vi "_s_Bronkhorst Serial Read Flows.vi"(6 "Delay Time (s)":dbl=0.1, 7 "Comunicaciones":T2={"Flujo_1"="COM1", "Brk1"=FALSE, "Flujo_2"="COM2", "Brk2"=FALSE, "Flujo_3"="COM3", "Brk3"=FALSE, "Flujo_4"="COM4", "Brk4"=FALSE, "Eurothe"="COM5", "Eurot"=FALSE, "Balanza"="ASRL6::INSTR", "Bal"=FALSE, "eValPos"="ASRL6::INSTR", "eVal"=FALSE, "flowbus"="ASRL6::INSTR", "fb"=FALSE}, 8 "error in (no error)":errorcluster) -> (0 "error out":errorcluster, 2 "Dispositivos":T1=[["3", "NO", "M0000013", "Air", "1", "ln/mn", "0", "0"], ["4", "NO", "M0000014", "Air", "1", "ln/mn", "0", "0"], ["5", "NO", "M0000015", "Air", "1", "ln/mn", "0", "0"], ["6", "NO", "M0000016", "Air", "1", "ln/mn", "0", "0"], ["7", "NO", "M0000017", "Air", "1", "ln/mn", "0", "0"], ["8", "NO", "M0000018", "Air", "1", "ln/mn", "0", "0"], ["9", "NO", "M0000019", "Air", "1", "ln/mn", "0", "0"], ["10", "NO", "M0000020", "Air", "1", "ln/mn", "0", "0"], ["11", "NO", "M0000021", "Air", "1", "ln/mn", "0", "0"]] caption="MassFlowControllers")   [LabVIEW 2013]
uses:
  Controles/P2018 Com Control.ctl
  _s_TablaBronkhorst.ctl
  _s_Bronkhorst Control.ctl
  P2022 TB INCAR GLOBALES.vi
panel:
  out "Num. of nodes":u32=6
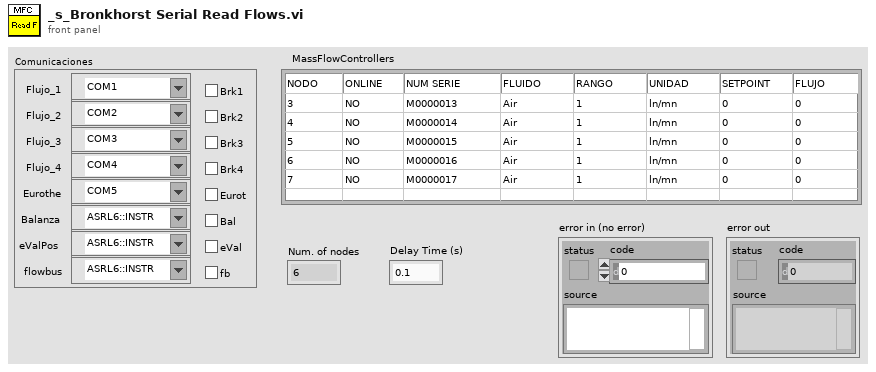
[diagram p1: front panel]
types:
  T1 = typedef "_s_TablaBronkhorst.ctl" = string[][]
  T2 = typedef "P2018 Com Control.ctl" = cluster{"Flujo_1":refnum<visa-resource-name>, "Brk1":bool, "Flujo_2":refnum<visa-resource-name>, "Brk2":bool, "Flujo_3":refnum<visa-resource-name>, "Brk3":bool, "Flujo_4":refnum<visa-resource-name>, "Brk4":bool, "Eurothe":refnum<visa-resource-name>, "Eurot":bool, "Balanza":refnum<visa-resource-name>, "Bal":bool, "eValPos":refnum<visa-resource-name>, "eVal":bool, "flowbus":refnum<visa-resource-name>, "fb":bool}
  T3 = typedef "P2018 Bronkhorst Control.ctl" = cluster{"Dispositivos":T1, "NuevosSP":string[][], "Nodes":u32, "Delay(s)":dbl}
  T4 = typedef "_s_Bronkhorst Control.ctl" = enum16{"Inicializar", "Request IdnString", "Request Serial Number", "Request Fluid Number", "Request Fluid Name", "Request Sensor Type", "Request Cap 0", "Request Cap100", "Request Units", "Request CapUnitStr", "Request Setpoint %", "Request Setpoint", "Request Measure %", "Request Measure ", "Send Control Mode", "Send Fluid Number", "Send Setpoint %", "Send Setpoint", "Shutdown"}
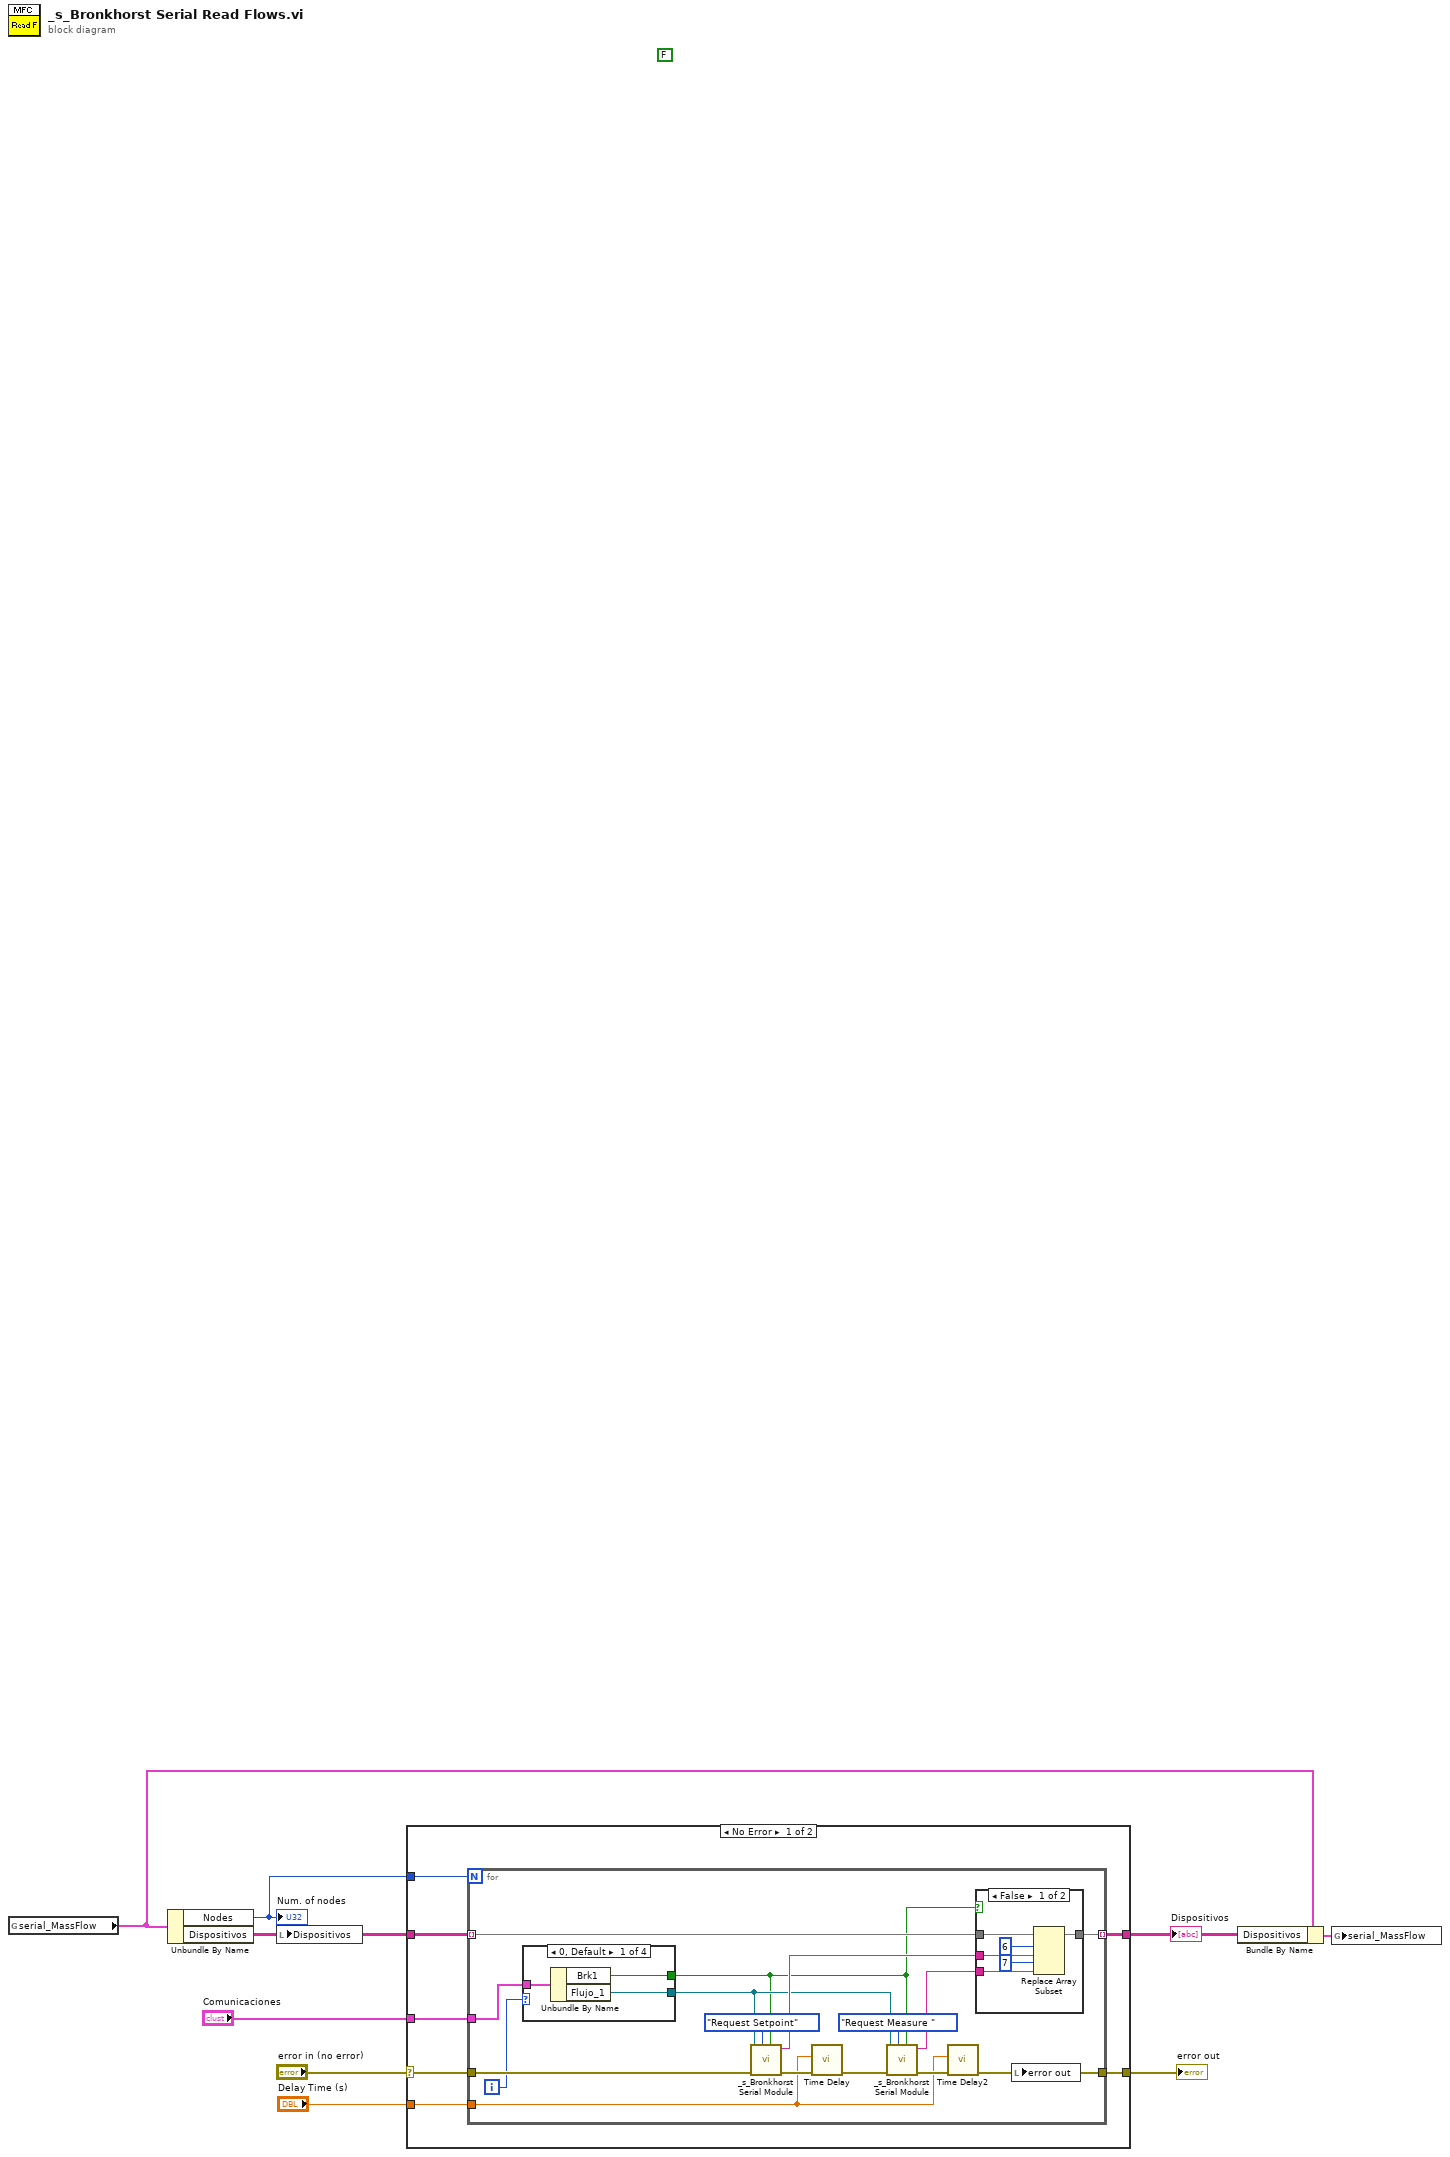
[diagram p0: block diagram]
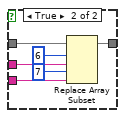
[diagram p2: hidden frame]
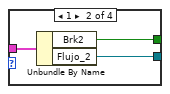
[diagram p3: hidden frame]
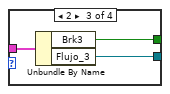
[diagram p4: hidden frame]
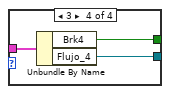
[diagram p5: hidden frame]
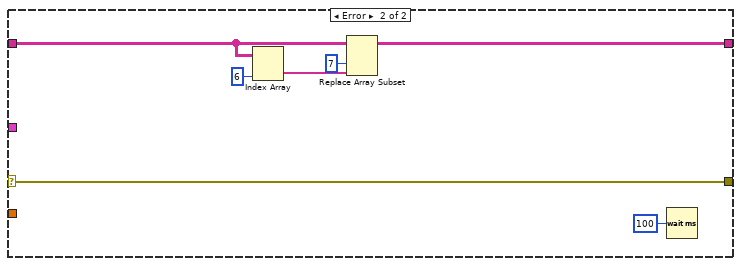
[diagram p6: hidden frame]
diagram:
  (unwired) FALSE
  n1 = global read "P2022 TB INCAR GLOBALES.vi" "serial_MassFlow"() -> (w9:T3)
  n2 = Unbundle By Name(w9) -> ("Nodes"=w4:u32, "Dispositivos"=w7:T1)
  "Num. of nodes" <- w4
  n3 = local write "Dispositivos"(w7) -> ()
  n4 = case shown="No Error" "error in (no error)" {
    selector: "error in (no error)" -> [w10 w57]
    tunnel: [w14 w60] -> w6
    tunnel: [w16 w57] -> w3
    tunnel: w7 -> [w15 w61]
    tunnel: "Delay Time (s)" -> [w13 _]
    tunnel: w4 -> [w12 _]
    tunnel: "Comunicaciones" -> [w11 _]
    frame No Error {
      n5 = for {
        N: w12 -> [_]
        tunnel: w10 -> [w25]
        tunnel: [w26] -> w16
        tunnel: w13 -> [w27]
        tunnel: w15 -> [w24] mode=indexing
        tunnel: [w23] -> w14 mode=indexing
        tunnel: w11 -> [w20]
        i -> [w19]
        n6 = case shown="0, Default" w19 {
          tunnel: w20 -> [w47 w50 w53 w56]
          tunnel: [w46 w49 w52 w55] -> w17
          tunnel: [w45 w48 w51 w54] -> w18
          frame 0, Default {
            n7 = Unbundle By Name(w47) -> ("Brk1"=w46:bool, "Flujo_1"=w45:refnum<visa-resource-name>)
          }
          frame 1 {
            n8 = Unbundle By Name(w50) -> ("Brk2"=w49:bool, "Flujo_2"=w48:refnum<visa-resource-name>)
          }
          frame 2 {
            n9 = Unbundle By Name(w53) -> ("Brk3"=w52:bool, "Flujo_3"=w51:refnum<visa-resource-name>)
          }
          frame 3 {
            n10 = Unbundle By Name(w56) -> ("Brk4"=w55:bool, "Flujo_4"=w54:refnum<visa-resource-name>)
          }
        }
        n11 = call "_s_Bronkhorst Serial Module.vi"("Module (T:Enable)"=w17, "Command"=_s_Bronkhorst_Control."Request Setpoint", "error in (no error)"=w25, "VISA resource name"=w18) -> ("error out"=w31:errorcluster, "Value"=w22:string)  [unwired: 4 in, 2 out]
        n12 = call "Time Delay"("error in (no error)"=w31, "Delay Time (s)"=w27) -> ("error out"=w28:errorcluster)  [unwired: 9 in]
        n13 = call "_s_Bronkhorst Serial Module.vi"("Module (T:Enable)"=w17, "Command"=_s_Bronkhorst_Control."Request Measure ", "error in (no error)"=w28, "VISA resource name"=w18) -> ("error out"=w29:errorcluster, "Value"=w21:string)  [unwired: 4 in, 2 out]
        n14 = call "Time Delay2"("error in (no error)"=w29, "Delay Time (s)"=w27) -> ("error out"=w26:errorcluster)  [unwired: 9 in]
        n15 = case shown="False" w17 {
          tunnel: w24 -> [w38 w44]
          tunnel: [w36 w41] -> w23
          tunnel: w22 -> [w34 w40]
          tunnel: w21 -> [w33 w39]
          frame False {
            n16 = Replace Array Subset(array=w38, new element #1=w34, index #1=6 ("index"), new element #2=w33, index #2=7 ("index")) -> (w36:string[])
          }
          frame True {
            n17 = Replace Array Subset(array=w44, new element #1=w40, index #1=6 ("index"), new element #2=w39, index #2=7 ("index")) -> (w41:string[])
          }
        }
        n18 = local write "error out"(w26) -> ()
      }
    }
    frame Error {
      n19 = Index Array(array=w61, index (col)=6 ("index")) -> (element=w62:string[])  [unwired: 1 in]
      n20 = Replace Array Subset(array=w61, new element=w62, index (col)=7 ("index")) -> (w60:T1)  [unwired: 1 in]
      n21 = Wait (ms)(milliseconds to wait=u32 100) -> ()  [unwired: 1 out]
    }
  }
  "Dispositivos" <- w6
  "error out" <- w3
  n22 = Bundle By Name(cluster=w9, "Dispositivos"=w6) -> (w5:T3)
  n23 = global write "P2022 TB INCAR GLOBALES.vi" "serial_MassFlow"(w5) -> ()
